vi "Unpack for gRPC.vi"(8 "error in":errorcluster, 9 "configuration / results":enum16{"Configuration", "Results"}(ring), 10 "any":T1, 11 "measurement customizations in":refnum<class "Measurement Plugin.lvclass">) -> (0 "error out":errorcluster, 2 "data value":variant, 3 "measurement customizations out":refnum<class "Measurement Plugin.lvclass">)   [LabVIEW 2024, in "Eff And Load Reg_Channel Ganging.lvlib" / "Measurement Plugin.lvclass"]
uses:
  Measurement Plugin.lvclass
  <vilib>/gRPC/LabVIEW gRPC Library/Shared/Any.ctl
  Measurement Configuration.ctl
  Measurement Results.ctl
  a521b266-ce99-437c-923d-067dcf1e07fd.vi
  3ecd018e-d556-4cbc-bc60-c4ba57204520.vi
  <vilib>/gRPC/LabVIEW gRPC Library/Server API/Translate Protobuf Error.vi
  <vilib>/AdvancedString/1D String Array to Delimited String.vi
  <vilib>/gRPC/LabVIEW gRPC Library/Server API/Server/Get Server DLL Path.vi
  Measurement Plugin.lvclass/Measurement Plugin.ctl
  Eff And Load Reg_Channel Ganging.lvlib
  <vilib>/Plug-In SDKs/Measurements/Measurement Plugin Service/Measurement Plugin Service.lvclass
  <vilib>/gRPC/LabVIEW gRPC Library/grpc-lvsupport-release.lvlib
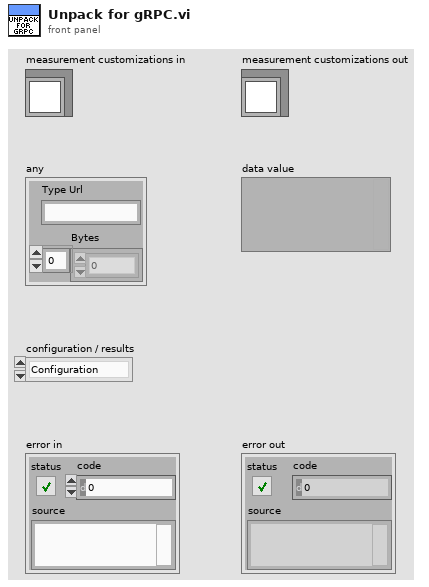
[diagram p1: front panel]
types:
  T1 = typedef "grpc-lvsupport-release.lvlib/Any.ctl" = cluster{"Type Url":string, "Bytes":u8[]}
  T2 = typedef "grpc-lvsupport-release.lvlib/grpcId.ctl" = u64
  T3 = typedef "Eff And Load Reg_Channel Ganging.lvlib/Measurement Configuration.ctl" = cluster{"Source master resource name":string, "Source slave resource names":string[], "Load master resource name":string, "Load slave resource names":string[], "Source system configuration":enum32{"Series", "Parallel", "Manual"}, "Source start voltage":dbl, "Source stop voltage":dbl, "Source voltage sweep points":i32, "Source voltage level range":dbl, "Source sense":i32, "Source limit symmetry":enum32{"Symmetric", "Asymmetric"}, "Source current limit range":dbl, "Source current limit low":dbl, "Source current limit high":dbl, "Source transient response":i32, "Source voltage gain bandwidth":dbl, "Source voltage compensation frequency":dbl, "Source voltage pole-zero ratio":dbl, "Load system configuration":enum32{"Series", "Parallel", "Manual"}, "Load start current":dbl, "Load stop current":dbl, "Load current sweep points/points per decade":i32, "Load sweep type":string, "Load current level range":dbl, "Load sense":i32, "Load limit symmetry":enum32{"Symmetric", "Asymmetric"}, "Load voltage limit range":dbl, "Load voltage limit low":dbl, "Load voltage limit high":dbl, "Load transient response":i32, "Load current gain bandwidth":dbl, "Load current compensation frequency":dbl, "Load current pole-zero ratio":dbl, "DUT setup time":dbl, "Source delay":dbl, "Aperture time":dbl, "Nominal output voltage":dbl, "Mode of operation":enum32{"Power on the DUT", "Perform measurement", "Power off the DUT"}, "Measurement timeout":dbl}
  T4 = typedef "Eff And Load Reg_Channel Ganging.lvlib/Measurement Results.ctl" = cluster{"Source sweep points":i32, "Load sweep points":i32, "Voltage values":dbl[], "Efficiency":dbl[], "Ganged load currents":dbl[], "Ganged load voltages":dbl[], "Load voltage deviation":dbl[], "Status":string, "Status (Load)":string, "Enabled Sources":string[], "Enabled Loads":string[]}
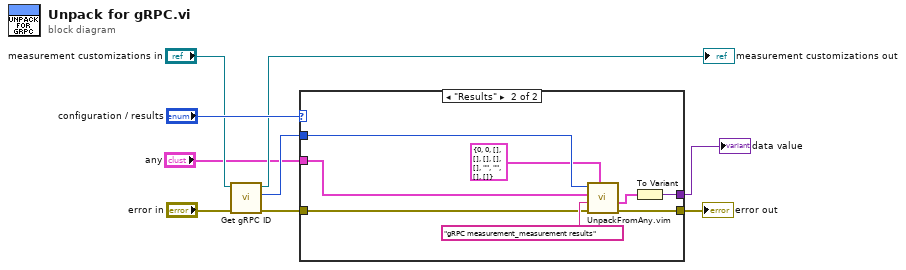
[diagram p0: block diagram]
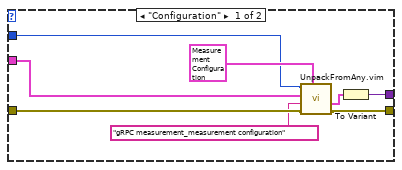
[diagram p2: hidden frame]
diagram:
  n1 = call <vilib>:"Get gRPC ID.vi"("error in"="error in", "measurement plugin service in"="measurement customizations in") -> ("error out"=w6:errorcluster, "gRPC ID"=w3:T2, "measurement plugin service out"=→"measurement customizations out":refnum<class "Measurement Plugin.lvclass">)  [unwired: 7 in]
  n2 = case shown="\"Results\"" "configuration / results" {
    tunnel: w6 -> [w15 w19]
    tunnel: "any" -> [w10 w18]
    tunnel: w3 -> [w12 w22]
    tunnel: [w16 w23] -> w9
    tunnel: [w17 w25] -> w1
    frame "Configuration" {
      n3 = call "UnpackFromAny.vim"("Data Type"=T3 {"Source master resource name"="", "Source slave resource names"=[], "Load master resource name"="", "Load slave resource names"=[], "Source system configuration"=enum."Parallel", "Source start voltage"=6.0, "Source stop voltage"=14.0, "Source voltage sweep points"=4, "Source voltage level range"=20.0, "Source sense"=1009, "Source limit symmetry"=enum."Asymmetric", "Source current limit range"=25.0, "Source current limit low"=-0.6, "Source current limit high"=25.0, "Source transient response"=1038, "Source voltage gain bandwidth"=2000.0, "Source voltage compensation frequency"=3530.0, "Source voltage pole-zero ratio"=2.0, "Load system configuration"=enum."Parallel", "Load start current"=1.0, "Load stop current"=50.0, "Load current sweep points/points per decade"=10, "Load sweep type"="Logarithmic", "Load current level range"=80.0, "Load sense"=1009, "Load limit symmetry"=enum."Symmetric", "Load voltage limit range"=6.0, "Load voltage limit low"=0.0, "Load voltage limit high"=inf, "Load transient response"=1038, "Load current gain bandwidth"=14000.0, "Load current compensation frequency"=180000.0, "Load current pole-zero ratio"=0.3, "DUT setup time"=1.0, "Source delay"=0.005, "Aperture time"=0.005, "Nominal output voltage"=1.0, "Mode of operation"=enum."Power on the DUT", "Measurement timeout"=0.0} ("Measurement Configuration"), "error in"=w15, "Message Type"="gRPC measurement_measurement configuration", "Any"=w10, "gRPCid in"=w12) -> ("error out"=w16:errorcluster, "Unpacked Value"=w14:T3)  [unwired: 4 in, 1 out]
      n4 = To Variant(anything=w14) -> (Variant=w17:variant)
    }
    frame "Results" {
      n5 = call "UnpackFromAny.vim"("Data Type"=T4 {"Source sweep points"=0, "Load sweep points"=0, "Voltage values"=[], "Efficiency"=[], "Ganged load currents"=[], "Ganged load voltages"=[], "Load voltage deviation"=[], "Status"="", "Status (Load)"="", "Enabled Sources"=[], "Enabled Loads"=[]} ("Measurement Results"), "error in"=w19, "Message Type"="gRPC measurement_measurement results", "Any"=w18, "gRPCid in"=w22) -> ("error out"=w23:errorcluster, "Unpacked Value"=w24:T4)  [unwired: 4 in, 1 out]
      n6 = To Variant(anything=w24) -> (Variant=w25:variant)
    }
  }
  "error out" <- w9
  "data value" <- w1
